vi "Init.vi"(8 "error in (no error)":errorcluster, 11 "dt":dbl) -> (0 "error out":errorcluster, 3 "Locus Recorder":refnum<class "Locus Recorder.lvclass">)   [LabVIEW 2013, in "Locus Recorder.lvclass"]
uses:
  Locus Recorder.lvclass
  Locus Recorder.lvclass/Locus Recorder.ctl
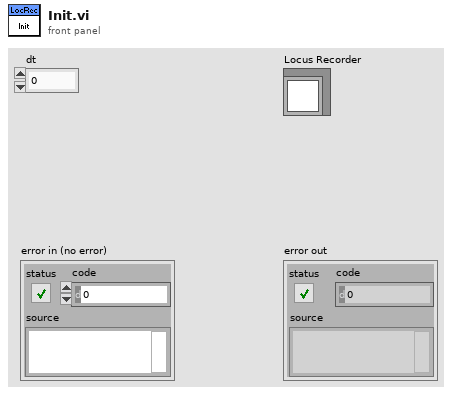
[diagram p1: front panel]
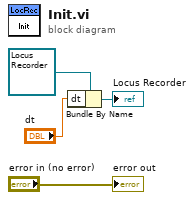
[diagram p0: block diagram]
diagram:
  n1 = Bundle By Name(cluster=refnum<class "Locus Recorder.lvclass"> refnum ("Locus Recorder.lvclass"), "dt"="dt") -> (→"Locus Recorder":refnum<class "Locus Recorder.lvclass">)
  "error out" <- "error in (no error)"
